vi "FTP自动升级更新main.vi"() -> ()   [LabVIEW 2016, in "自动更新.lvlib"]
uses:
  <vilib>/FTP/NI_FTP.lvlib
panel:
  out "有新版本":bool
  out "最新版本获取进度":u8(slide) scale=0.0..100.0
  # "版本获取中，请稍后！"
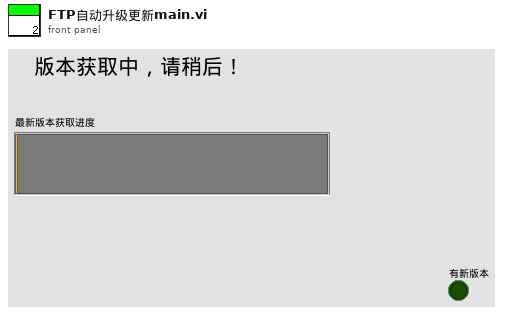
[diagram p1: front panel]
types:
  T1 = enum16{"get version information", "get success", "contact", "over"}
  T2 = cluster{"网络灯":bool, "接收中":bool, "已接收百分比":u8, "接收成功次数":dbl, "当前步骤":enum16{"init", "receivehead", "receivecontent", "receivesuccess", "over"}, "文件名":string, "error out":errorcluster}
  T3 = enum16{"open", "replace", "create", "open or create", "replace or create", "replace or create with confirmation"}
  T4 = cluster{"主机":string, "用户":string, "密码":string, "远程路径":string, "下载文件名":string, "软件版本":string}
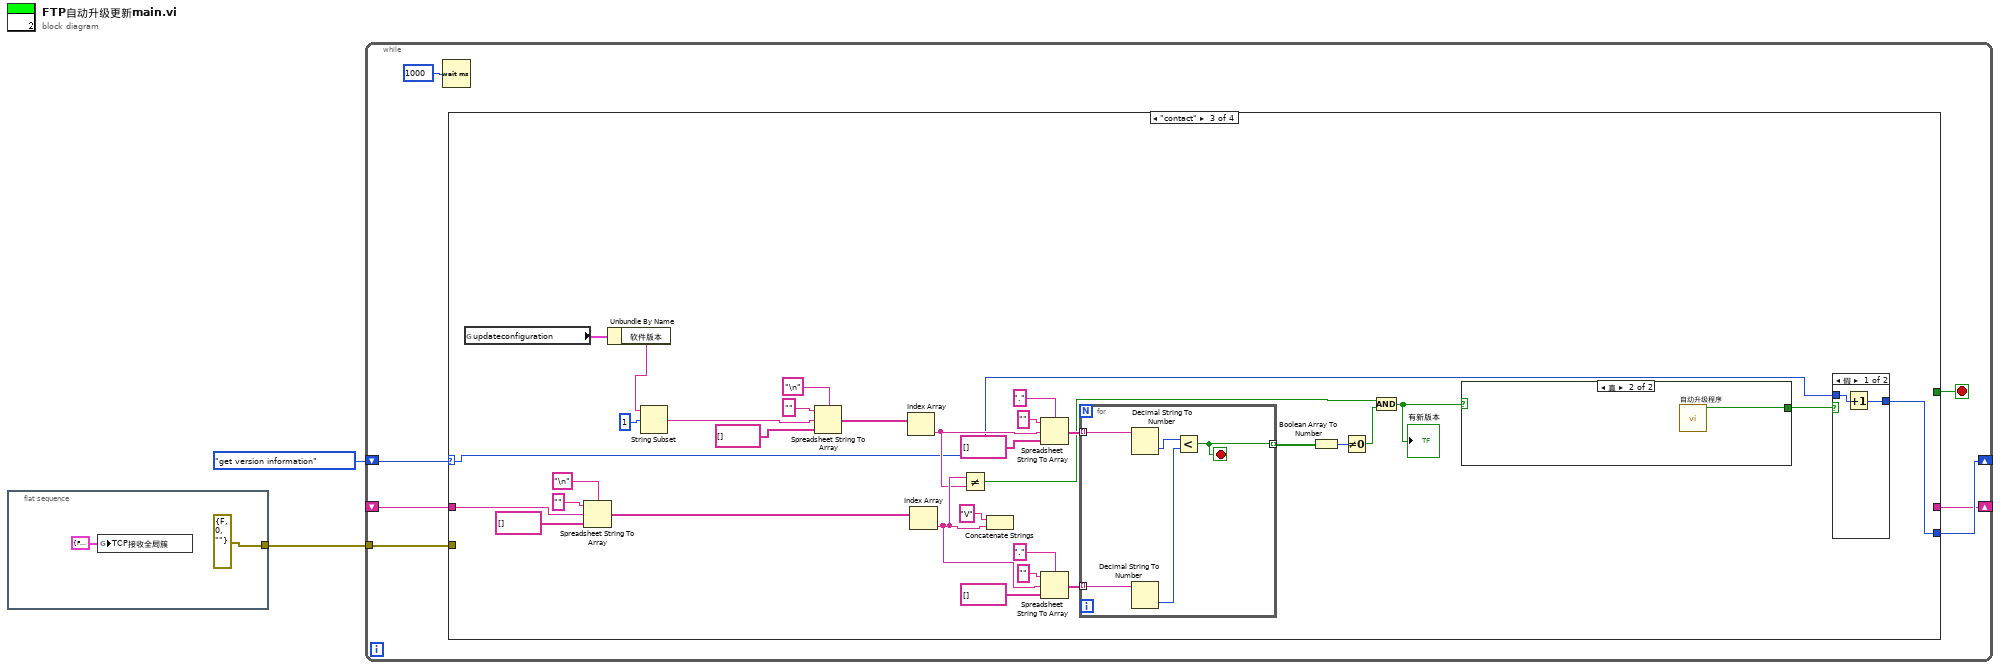
[diagram p0: block diagram]
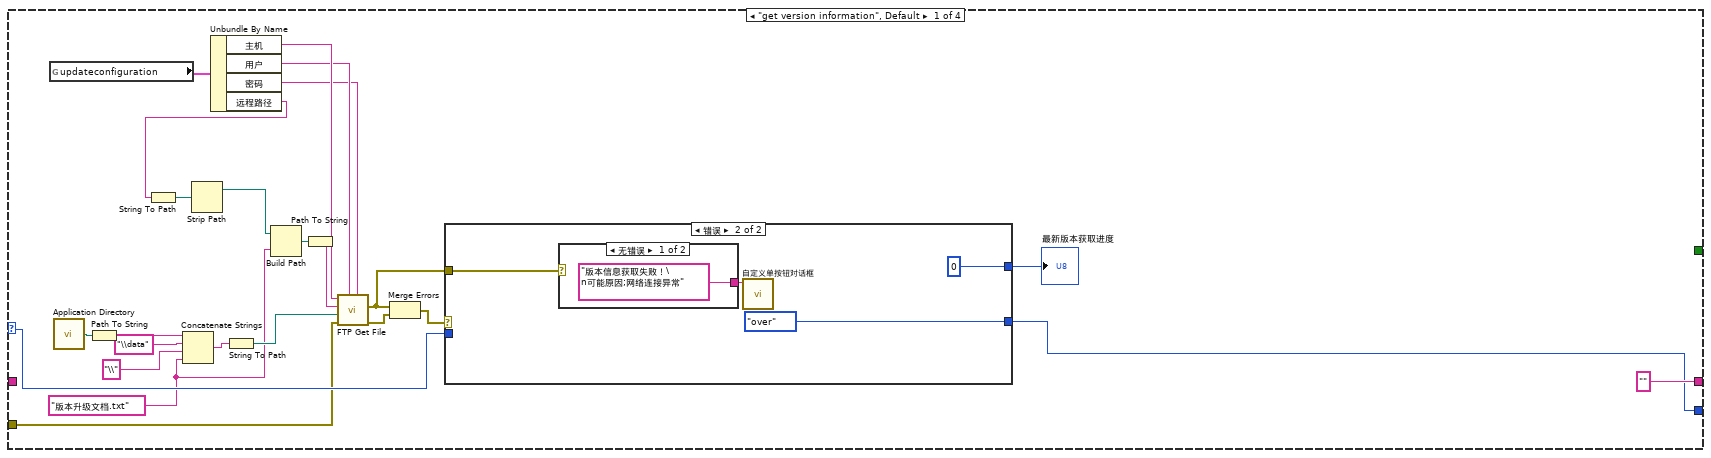
[diagram p2: hidden frame]
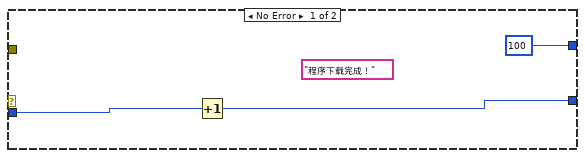
[diagram p3: hidden frame]
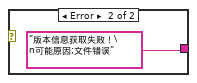
[diagram p4: hidden frame]
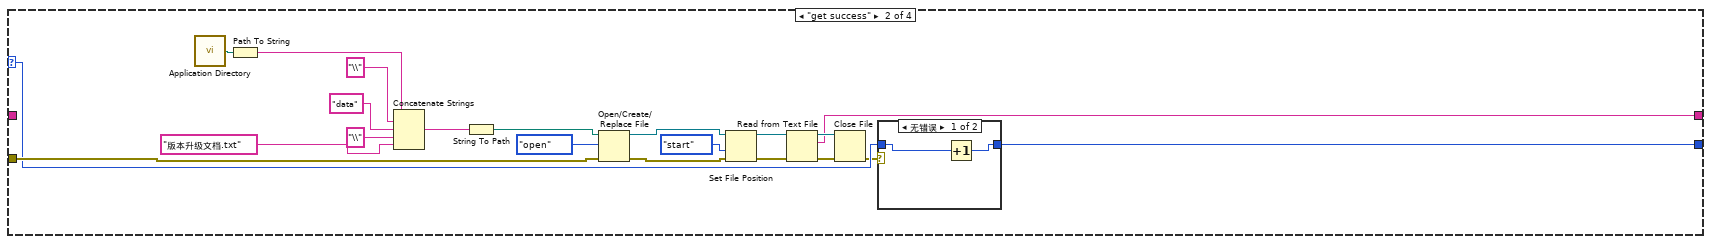
[diagram p5: hidden frame]
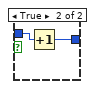
[diagram p7: hidden frame]
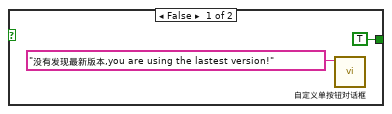
[diagram p8: hidden frame]
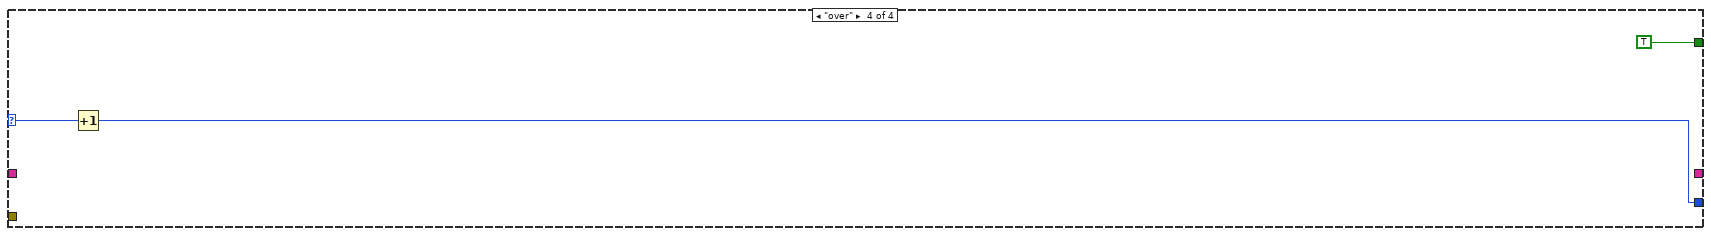
[diagram p9: hidden frame]
diagram:
  n1 = flat-sequence {
    tunnel: [errorcluster {"status"=FALSE, "code"=0, "source"=""} ("错误常量")] -> w1
    frame #0 {
      n2 = global write "全局变量1.vi" "TCP接收全局簇"(T2 {"网络灯"=FALSE, "接收中"=FALSE, "已接收百分比"=0, "接收成功次数"=0.0, "当前步骤"=enum."init", "文件名"="", "error out"={"status"=FALSE, "code"=0, "source"=""}} ("TCP接收全局簇")) -> ()
    }
  }
  n3 = while {
    shift-right: [w9] -> _
    shift-left: T1."get version information" -> [w10]
    tunnel: w1 -> [w8]
    shift-right: [w7] -> _
    shift-left: _ -> [w6]
    stop <- w5 stop-if-true
    n4 = Wait (ms)(milliseconds to wait=u32 1000 ("等待时间（毫秒）")) -> ()  [unwired: 1 out]
    n5 = case shown="\"contact\"" w10 {
      selector: w10 -> [w25 w52 w72 w114]
      tunnel: [w24 w51 w71 w113] -> w9
      tunnel: w8 -> [w23 w53 _ _]
      tunnel: ["" w45 _ _] -> w7
      tunnel: w6 -> [_ _ w75 _]
      tunnel: [_ _ _ TRUE] -> w5
      frame "get version information", Default {
        w14 = "版本升级文档.txt"
        n6 = global read "update全局.vi" "updateconfiguration"() -> (w22:T4)
        n7 = call <vilib>:"Application Directory.vi"() -> ("Application Directory"=w32:path)
        n8 = Path To String(path=w32) -> (string=w34:string)
        n9 = Concatenate Strings(w34, "\\data" ("字符串"), "\\" ("字符串"), w14) -> (w31:string)
        n10 = Unbundle By Name(w22) -> ("主机"=w21:string, "用户"=w20:string, "密码"=w19:string, "远程路径"=w15:string)
        n11 = String To Path(string=w15) -> (path=w17:path)
        n12 = Strip Path(path=w17) -> (stripped path=w16:path)  [unwired: 1 out]
        n13 = String To Path(string=w31) -> (path=w30:path)
        n14 = Build Path(base path=w16, name or relative path=w14) -> (appended path=w13:path)
        n15 = Path To String(path=w13) -> (string=w12:string)
        n16 = call <vilib>:"FTP Get File.vi"("password"=w19, "user"=w20, "error in (no error)"=w23, "local path"=w30, "remote path"=w12, "host"=w21) -> ("error out"=w29:errorcluster, "file error"=w27:errorcluster)  [unwired: 4 in]
        n17 = Merge Errors(w27, w29) -> (w28:errorcluster)
        n18 = case shown="错误" w28 {
          tunnel: w27 -> [_ w41]
          tunnel: [u8 100 ("y") u8 0 ("y")] -> w26
          tunnel: [w37 T1."over"] -> w24
          tunnel: w25 -> [w36 _]
          frame No Error {
            (unwired) "程序下载完成！"
            n19 = Increment(x=w36) -> (x+1=w37:T1)
          }
          frame Error {
            n20 = case shown="无错误" w41 {
              tunnel: ["版本信息获取失败！\n可能原因;网络连接异常" "版本信息获取失败！\n可能原因;文件错误"] -> w42
              frame No Error {
              }
              frame Error {
              }
            }
            n21 = call "自定义单按钮对话框.vi"("消息"=w42) -> ()  [unwired: 11 in]
          }
        }
        "最新版本获取进度" <- w26
      }
      frame "get success" {
        n22 = call <vilib>:"Application Directory.vi"() -> ("Application Directory"=w58:path)
        n23 = Path To String(path=w58) -> (string=w61:string)
        n24 = Concatenate Strings(w61, "\\" ("字符串"), "data" ("字符串"), "\\" ("字符串"), "版本升级文档.txt" ("字符串")) -> (w55:string)
        n25 = String To Path(string=w55) -> (path=w54:path)
        n26 = Open/Create/Replace File(file path (use dialog)=w54, error in=w53, operation (0:open)=T3."open" ("操作(0:open)")) -> (refnum out=w64:refnum<file>, error out=w63:errorcluster)  [unwired: 3 in, 1 out]
        n27 = Set File Position(refnum=w64, from (0:start)=enum16{"start", "end", "current"}."start" ("自（0:起始）"), error in=w63) -> (refnum out=w49:refnum<file>, error out=w48:errorcluster)  [unwired: 1 in]
        n28 = Read from Text File(file (use dialog)=w49, error in=w48) -> (refnum out=w50:refnum<file>, text=w45:string, error out=w47:errorcluster)  [unwired: 2 in, 1 out]
        n29 = Close File(refnum=w50, error in=w47) -> (error out=w46:errorcluster)  [unwired: 1 out]
        n30 = case shown="无错误" w46 {
          tunnel: w52 -> [w67 w68]
          tunnel: [w66 w68] -> w51
          frame No Error {
            n31 = Increment(x=w67) -> (x+1=w66:T1)
          }
          frame Error {
          }
        }
      }
      frame "contact" {
        n32 = global read "update全局.vi" "updateconfiguration"() -> (w70:T4)
        n33 = Spreadsheet String To Array(delimiter (Tab)="\n" ("分隔符(Tab)"), format string="" ("格式字符串"), spreadsheet string=w75, array type (2D Dbl)=string[] []) -> (array=w96:string[])
        n34 = Unbundle By Name(w70) -> ("软件版本"=w69:string)
        n35 = String Subset(string=w69, offset (0)=1 ("偏移量(0)")) -> (substring=w88:string)  [unwired: 1 in]
        n36 = Spreadsheet String To Array(delimiter (Tab)="\n" ("分隔符(Tab)"), format string="" ("格式字符串"), spreadsheet string=w88, array type (2D Dbl)=string[] []) -> (array=w87:string[])
        n37 = Index Array(array=w87) -> (element=w78:string)  [unwired: 1 in]
        n38 = Index Array(array=w96) -> (element=w79:string)  [unwired: 1 in]
        n39 = Not Equal?(x=w79, y=w78) -> (x != y?=w76:bool)
        n40 = Concatenate Strings("V" ("字符串"), w79) -> ()  [unwired: 1 out]
        n41 = Spreadsheet String To Array(delimiter (Tab)="." ("分隔符(Tab)"), format string="" ("格式字符串"), spreadsheet string=w78, array type (2D Dbl)=string[] []) -> (array=w82:string[])
        n42 = Spreadsheet String To Array(delimiter (Tab)="." ("分隔符(Tab)"), format string="" ("格式字符串"), spreadsheet string=w79, array type (2D Dbl)=string[] []) -> (array=w83:string[])
        n43 = for {
          tunnel: w83 -> [w110] mode=indexing
          tunnel: w82 -> [w112] mode=indexing
          tunnel: [w111] -> w81 mode=indexing
          stop <- w111 stop-if-true
          n44 = Decimal String To Number(string=w112) -> (number=w109:i32)  [unwired: 2 in, 1 out]
          n45 = Decimal String To Number(string=w110) -> (number=w108:i32)  [unwired: 2 in, 1 out]
          n46 = Less?(x=w109, y=w108) -> (x < y?=w111:bool)
        }
        n47 = Boolean Array To Number(Boolean array=w81) -> (number=w80:u32)
        n48 = Not Equal To 0?(x=w80) -> (x != 0?=w77:bool)
        n49 = And(x=w76, y=w77) -> (x .and. y?=w74:bool)
        "有新版本" <- w74
        n50 = case shown="真" w74 {
          tunnel: [TRUE ("确定") w107] -> w73
          frame False {
            n51 = call "自定义单按钮对话框.vi"("消息"="没有发现最新版本,you are using the lastest version!") -> ()  [unwired: 11 in]
          }
          frame True {
            n52 = call "自动升级程序.vi"() -> ("确定"=w107:bool)  [unwired: 10 in, 1 out]
          }
        }
        n53 = case shown="假" w73 {
          tunnel: w72 -> [w102 w104]
          tunnel: [w101 w103] -> w71
          frame False {
            n54 = Increment(x=w102) -> (x+1=w101:T1)
          }
          frame True {
            n55 = Increment(x=w104) -> (x+1=w103:T1)
          }
        }
      }
      frame "over" {
        n56 = Increment(x=w114) -> (x+1=w113:T1)
      }
    }
  }
